vi "BASE-Main.vi"() -> ()   [LabVIEW 2017]
uses:
  <vilib>/Utility/error.llb/DialogType.ctl
  55ed0eea-cd20-493f-8468-85b8c1a0a0c0.vi
panel:
  in  "RECIPE":bool
  out "error out":errorcluster
  in  "Logout":bool
  in  "Stop":bool
  in  "Create Login":bool
  in  "Reports":bool
  in  "Start":bool
  out "Time":string
  out "Date":string
  in  "Login":bool
  # "USB CONNECTOR TESTING"
types:
  T1 = enum8{"Enabled", "Disabled", "Disabled and Grayed Out"}
  T2 = typedef "DialogType.ctl" = u16
  T3 = enum32{"Invalid", "Standard", "Closed", "Hidden", "Minimized", "Maximized"}
  T4 = enum32{"invalid app kind", "Development System", "Run Time System", "Student Edition", "Embedded LabVIEW", "Evaluation", "Custom"}
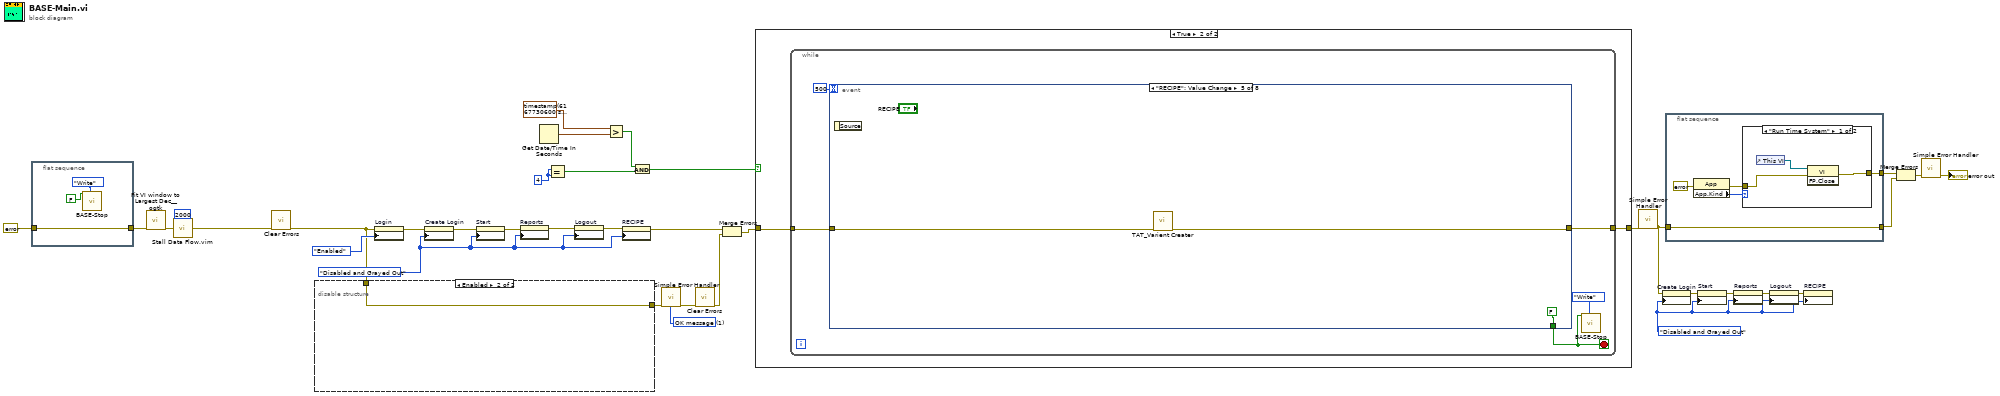
[diagram p0: block diagram]
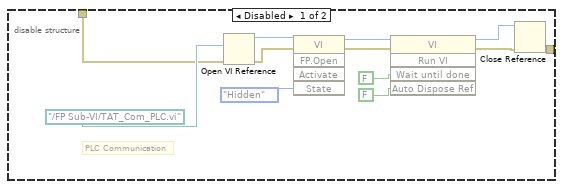
[diagram p2: hidden frame]
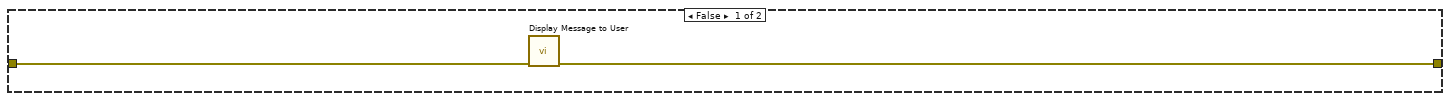
[diagram p4: hidden frame]
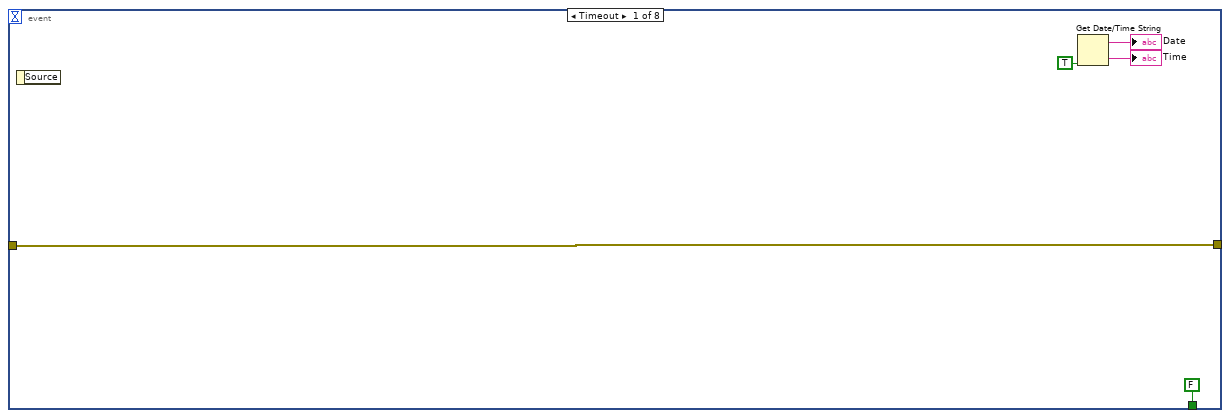
[diagram p5: hidden frame]
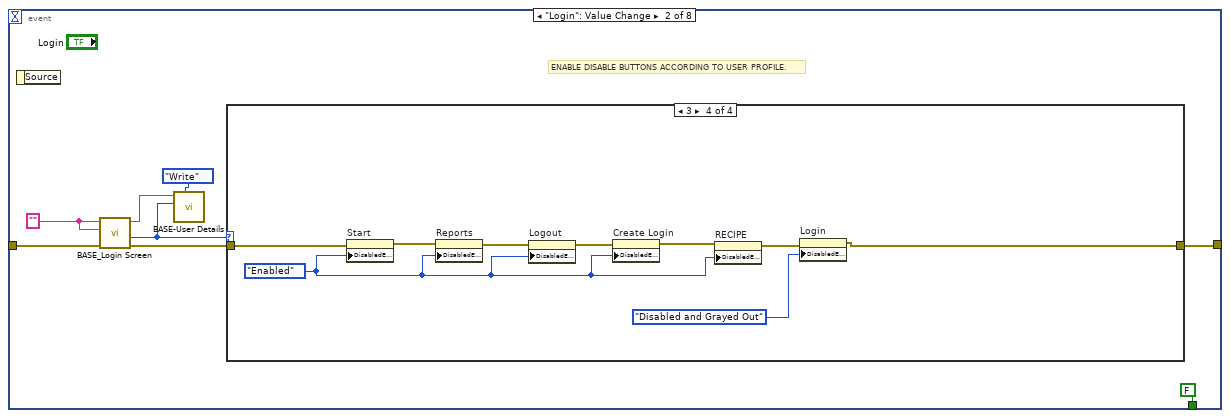
[diagram p6: hidden frame]
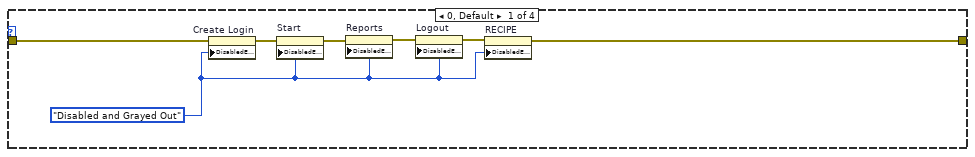
[diagram p7: hidden frame]
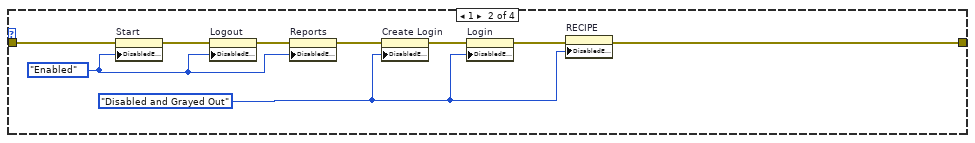
[diagram p8: hidden frame]
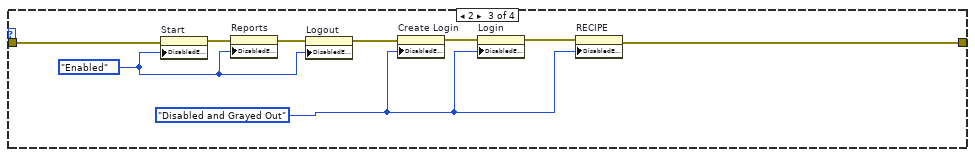
[diagram p9: hidden frame]
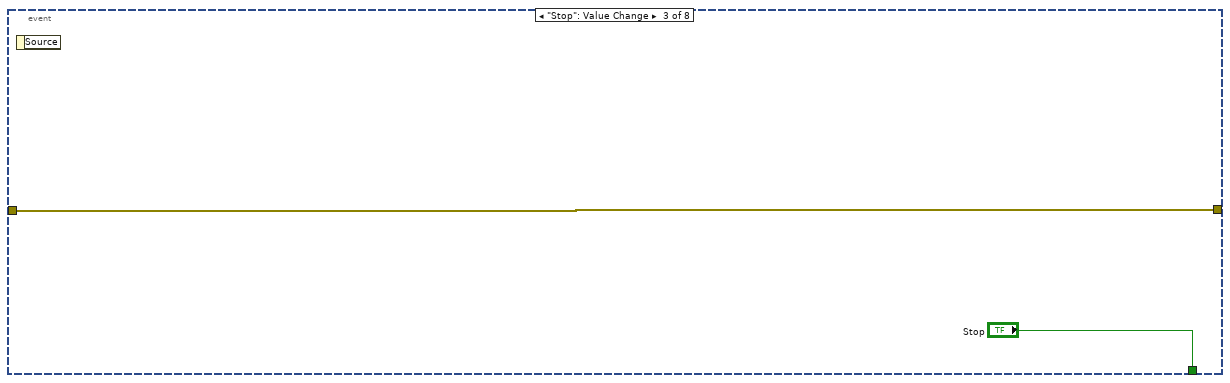
[diagram p10: hidden frame]
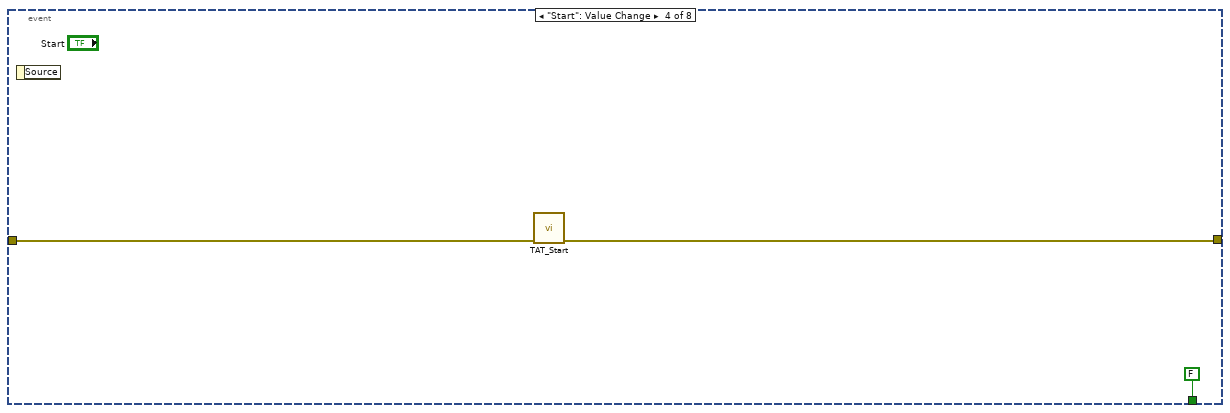
[diagram p11: hidden frame]
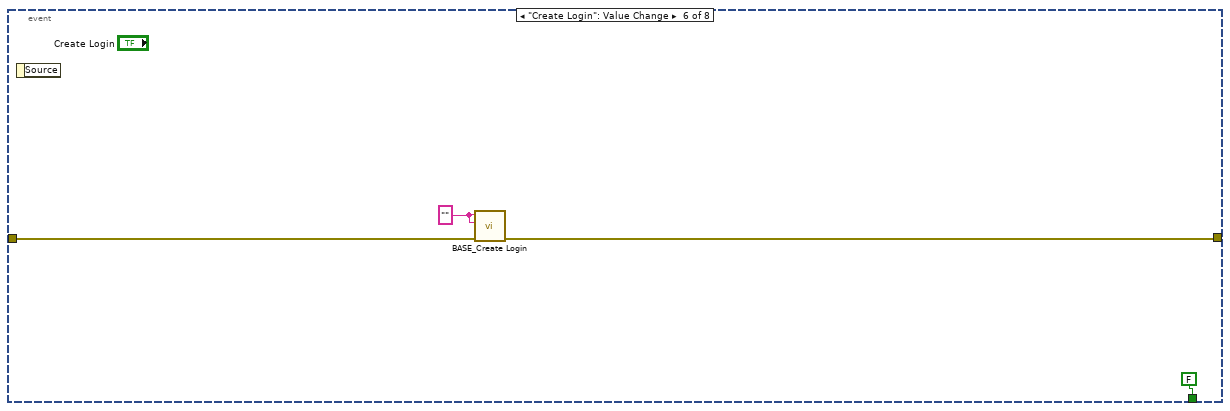
[diagram p12: hidden frame]
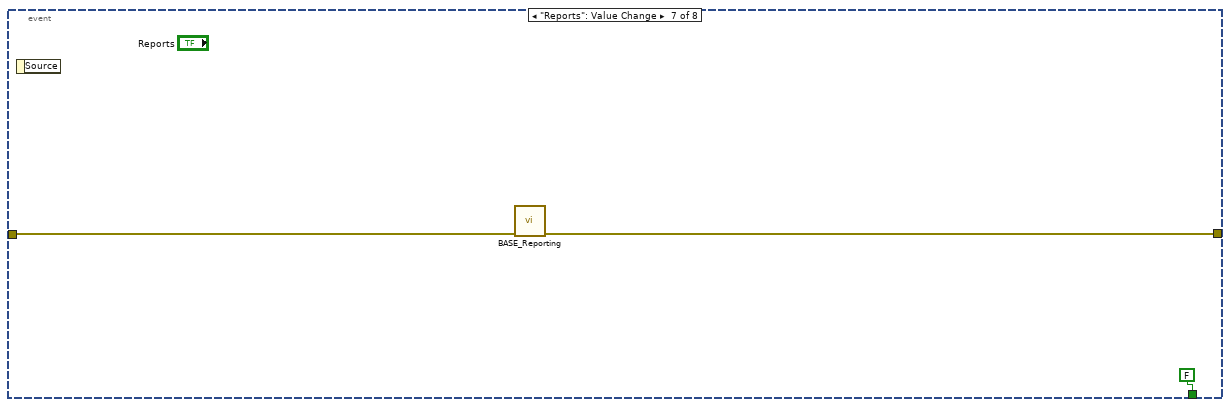
[diagram p13: hidden frame]
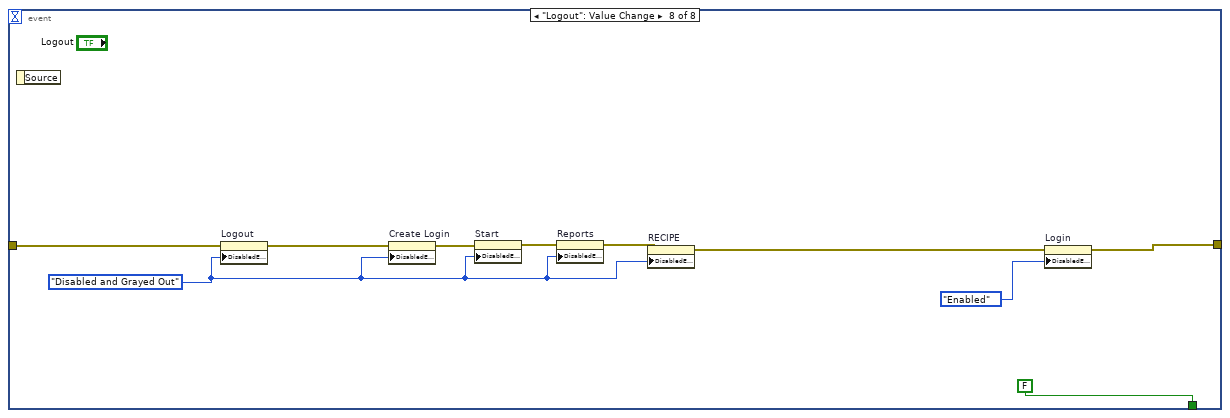
[diagram p14: hidden frame]
diagram:
  w8 = T1."Disabled and Grayed Out" ("Disabled")
  w1 = 4 ("y")
  w24 = T2 1 items=["no dialog", "OK message", "continue or stop message", "OK message + warnings", "continue/stop + warnings"] ("type of dialog (OK msg:1)")
  w9 = T1."Disabled and Grayed Out" ("Disabled")
  n1 = flat-sequence {
    tunnel: [w39] -> w27
    tunnel: errorcluster {"status"=FALSE, "code"=0, "source"=""} ("error constant") -> [w39]
    frame #0 {
      n2 = call "BASE-Stop.vi"("Enum"=enum16{"Read", "Write"}."Write", "Stop"=FALSE) -> ()  [unwired: 9 in, 1 out]
    }
  }
  n3 = call <userlib>:"Fit VI window to Largest Dec__ogtk.vi"("error in (no error)"=w27) -> ("error out"=w14:errorcluster)  [unwired: 5 in, 1 out]
  n4 = call "Stall Data Flow.vim"("value in"=w14, "milliseconds to wait"=u32 2000) -> ("value out"=w13:errorcluster)  [unwired: 1 out]
  n5 = call <vilib>:"Clear Errors.vi"("error in (no error)"=w13) -> ("error out"=w20:errorcluster)  [unwired: 5 in, 1 out]
  n6 = disable-structure shown="Enabled" {
    disable-tunnel: [w41 w52] -> w25
    disable-tunnel: w20 -> [w40 w52]
    frame Disabled {
      # "PLC Communication"
      n7 = Open VI Reference(vi path=path "../FP Sub-VI/TAT_Com_PLC.vi", error in (no error)=w40) -> (vi reference=w48:refnum<vi>, error out=w49:errorcluster)  [unwired: 4 in]
      n8 = invoke class="VI" method="FP.Open"(reference=w48, error in=w49, "State"=T3."Hidden") -> (reference out=w51:refnum<vi>, error out=w50:errorcluster)  [unwired: 2 in, 3 out]
      n9 = invoke class="VI" method="Run VI"(reference=w51, error in=w50, "Wait until done"=FALSE ("Wait Until Done"), "Auto Dispose Ref"=FALSE ("Auto Dispose Reference")) -> (reference out=w47:refnum<vi>, error out=w46:errorcluster)  [unwired: 1 in, 3 out]
      n10 = Close Reference(reference=w47, error in (no error)=w46) -> (error out=w41:errorcluster)
    }
    frame Enabled {
    }
  }
  n11 = property on="Login" class="Bool"(error in=w20, "DisabledEnum"=T1."Enabled" ("Disabled")) -> (error out=w31:errorcluster)  [unwired: 1 in, 1 out]
  n12 = property on="Create Login" class="Bool"(error in=w31, "DisabledEnum"=w9) -> (error out=w35:errorcluster)  [unwired: 1 in, 1 out]
  n13 = property on="Start" class="Bool"(error in=w35, "DisabledEnum"=w9) -> (error out=w10:errorcluster)  [unwired: 1 in, 1 out]
  n14 = property on="Reports" class="Bool"(error in=w10, "DisabledEnum"=w9) -> (error out=w29:errorcluster)  [unwired: 1 in, 1 out]
  n15 = Get Date/Time In Seconds() -> (seconds since 1Jan1904=w16:timestamp)
  n16 = Equal?(x=w1, y=w1) -> (x = y?=w19:bool)
  n17 = property on="Logout" class="Bool"(error in=w29, "DisabledEnum"=w9) -> (error out=w11:errorcluster)  [unwired: 1 in, 1 out]
  n18 = Greater?(x=timestamp(6167730600 s since 1904-01-01), y=w16) -> (0:w15:bool)
  n19 = property on="RECIPE" class="Bool"(error in=w11, "DisabledEnum"=w9) -> (error out=w2:errorcluster)  [unwired: 1 in, 1 out]
  n20 = And(x=w15, y=w19) -> (x .and. y?=w18:bool)
  n21 = call <vilib>:"Simple Error Handler.vi"("type of dialog (OK msg:1)"=w24, "error in (no error)"=w25) -> ("error out"=w23:errorcluster)  [unwired: 3 in, 4 out]
  n22 = call <vilib>:"Clear Errors.vi"("error in (no error)"=w23) -> ("error out"=w22:errorcluster)  [unwired: 5 in, 1 out]
  n23 = Merge Errors(w2, w22) -> (w26:errorcluster)
  n24 = case shown="True" w18 {
    tunnel: w26 -> [w54 w56]
    tunnel: [w53 w55] -> w36
    frame False {
      n25 = call "Display Message to User"("error in (no error)"=w54) -> ("error out"=w53:errorcluster)  [unwired: 9 in, 1 out]
    }
    frame True {
      n26 = while {
        tunnel: w56 -> [w60]
        tunnel: [w59] -> w55
        stop <- w57 stop-if-true
        n27 = event shown="[4] \"RECIPE\": Value Change" {
          selector: _ -> [_ _ _ _ _ _ _ _]
          dyn-events: _ -> [_ _ _ _ _ _ _ _]
          timeout: 500 -> [_ _ _ _ _ _ _ _]
          tunnel: w60 -> [w64 w74 w109 w112 w115 w120 w122 w130]
          tunnel: [w64 w67 w109 w111 w114 w119 w121 w131] -> w59
          tunnel: [FALSE ("Stop") FALSE ("Stop") "Stop" FALSE ("Stop") FALSE ("Stop") FALSE ("Stop") FALSE ("Stop") FALSE ("Stop")] -> w57
          event Timeout {
            n28 = event-data() -> ()  [unwired: 1 in, 1 out]
            n29 = Get Date/Time String(want seconds? (F)=TRUE) -> (date string=→"Date":string, time string=→"Time":string)  [unwired: 2 in]
          }
          event "Login": Value Change {
            w70 = "" ("User Name")
            # "ENABLE DISABLE BUTTONS ACCORDING TO USER PROFILE."
            n30 = event-data() -> ()  [unwired: 1 in, 1 out]
            n31 = call "BASE_Login Screen.vi"("Error In"=w74, "Password"=w70, "User Name"=w70) -> ("error out"=w73:errorcluster, "Level"=w68:i32, "User Name Out"=w71:string)  [unwired: 5 in, 1 out]
            n32 = call "BASE-User Details.vi"("Enum"=enum16{"Read", "Write"}."Write", "Level In"=w68, "User Name In"=w71) -> ()  [unwired: 7 in, 2 out]
            n33 = case shown="3" w68 {
              tunnel: w73 -> [w79 w90 w99 w108]
              tunnel: [w75 w82 w91 w100] -> w67
              frame 0, Default {
                w76 = T1."Disabled and Grayed Out" ("Disabled")
                n34 = property on="Create Login" class="Bool"(error in=w79, "DisabledEnum"=w76) -> (error out=w81:errorcluster)  [unwired: 1 in, 1 out]
                n35 = property on="Start" class="Bool"(error in=w81, "DisabledEnum"=w76) -> (error out=w80:errorcluster)  [unwired: 1 in, 1 out]
                n36 = property on="Reports" class="Bool"(error in=w80, "DisabledEnum"=w76) -> (error out=w77:errorcluster)  [unwired: 1 in, 1 out]
                n37 = property on="Logout" class="Bool"(error in=w77, "DisabledEnum"=w76) -> (error out=w78:errorcluster)  [unwired: 1 in, 1 out]
                n38 = property on="RECIPE" class="Bool"(error in=w78, "DisabledEnum"=w76) -> (error out=w75:errorcluster)  [unwired: 1 in, 1 out]
              }
              frame 1 {
                w84 = T1."Disabled and Grayed Out" ("Disabled")
                w83 = T1."Enabled" ("Disabled")
                n39 = property on="Start" class="Bool"(error in=w90, "DisabledEnum"=w83) -> (error out=w86:errorcluster)  [unwired: 1 in, 1 out]
                n40 = property on="Logout" class="Bool"(error in=w86, "DisabledEnum"=w83) -> (error out=w88:errorcluster)  [unwired: 1 in, 1 out]
                n41 = property on="Reports" class="Bool"(error in=w88, "DisabledEnum"=w83) -> (error out=w89:errorcluster)  [unwired: 1 in, 1 out]
                n42 = property on="Create Login" class="Bool"(error in=w89, "DisabledEnum"=w84) -> (error out=w87:errorcluster)  [unwired: 1 in, 1 out]
                n43 = property on="Login" class="Bool"(error in=w87, "DisabledEnum"=w84) -> (error out=w85:errorcluster)  [unwired: 1 in, 1 out]
                n44 = property on="RECIPE" class="Bool"(error in=w85, "DisabledEnum"=w84) -> (error out=w82:errorcluster)  [unwired: 1 in, 1 out]
              }
              frame 2 {
                w92 = T1."Disabled and Grayed Out" ("Disabled")
                w93 = T1."Enabled" ("Disabled")
                n45 = property on="Start" class="Bool"(error in=w99, "DisabledEnum"=w93) -> (error out=w96:errorcluster)  [unwired: 1 in, 1 out]
                n46 = property on="Reports" class="Bool"(error in=w96, "DisabledEnum"=w93) -> (error out=w98:errorcluster)  [unwired: 1 in, 1 out]
                n47 = property on="Logout" class="Bool"(error in=w98, "DisabledEnum"=w93) -> (error out=w94:errorcluster)  [unwired: 1 in, 1 out]
                n48 = property on="Create Login" class="Bool"(error in=w94, "DisabledEnum"=w92) -> (error out=w97:errorcluster)  [unwired: 1 in, 1 out]
                n49 = property on="Login" class="Bool"(error in=w97, "DisabledEnum"=w92) -> (error out=w95:errorcluster)  [unwired: 1 in, 1 out]
                n50 = property on="RECIPE" class="Bool"(error in=w95, "DisabledEnum"=w92) -> (error out=w91:errorcluster)  [unwired: 1 in, 1 out]
              }
              frame 3 {
                w101 = T1."Enabled" ("Disabled")
                n51 = property on="Start" class="Bool"(error in=w108, "DisabledEnum"=w101) -> (error out=w103:errorcluster)  [unwired: 1 in, 1 out]
                n52 = property on="Reports" class="Bool"(error in=w103, "DisabledEnum"=w101) -> (error out=w107:errorcluster)  [unwired: 1 in, 1 out]
                n53 = property on="Logout" class="Bool"(error in=w107, "DisabledEnum"=w101) -> (error out=w106:errorcluster)  [unwired: 1 in, 1 out]
                n54 = property on="Create Login" class="Bool"(error in=w106, "DisabledEnum"=w101) -> (error out=w105:errorcluster)  [unwired: 1 in, 1 out]
                n55 = property on="RECIPE" class="Bool"(error in=w105, "DisabledEnum"=w101) -> (error out=w104:errorcluster)  [unwired: 1 in, 1 out]
                n56 = property on="Login" class="Bool"(error in=w104, "DisabledEnum"=T1."Disabled and Grayed Out" ("Disabled")) -> (error out=w100:errorcluster)  [unwired: 1 in, 1 out]
              }
            }
          }
          event "Stop": Value Change {
            n57 = event-data() -> ()  [unwired: 1 in, 1 out]
          }
          event "Start": Value Change {
            n58 = event-data() -> ()  [unwired: 1 in, 1 out]
            n59 = call "TAT_Start.vi"("error In"=w112) -> ("error out"=w111:errorcluster)  [unwired: 10 in]
          }
          event "RECIPE": Value Change {
            n60 = event-data() -> ()  [unwired: 1 in, 1 out]
            n61 = call "TAT_Varient Creater.vi"("error in (no error)"=w115) -> ("error out"=w114:errorcluster)  [unwired: 10 in]
          }
          event "Create Login": Value Change {
            w118 = "" ("User Name")
            n62 = event-data() -> ()  [unwired: 1 in, 1 out]
            n63 = call "BASE_Create Login.vi"("Error In"=w120, "Password"=w118, "User Name"=w118) -> ("error out"=w119:errorcluster)  [unwired: 6 in]
          }
          event "Reports": Value Change {
            n64 = event-data() -> ()  [unwired: 1 in, 1 out]
            n65 = call "BASE_Reporting.vi"("error in (no error)"=w122) -> ("error out"=w121:errorcluster)  [unwired: 10 in]
          }
          event "Logout": Value Change {
            w125 = T1."Disabled and Grayed Out" ("Disabled")
            n66 = event-data() -> ()  [unwired: 1 in, 1 out]
            n67 = property on="Logout" class="Bool"(error in=w130, "DisabledEnum"=w125) -> (error out=w126:errorcluster)  [unwired: 1 in, 1 out]
            n68 = property on="Create Login" class="Bool"(error in=w126, "DisabledEnum"=w125) -> (error out=w133:errorcluster)  [unwired: 1 in, 1 out]
            n69 = property on="Start" class="Bool"(error in=w133, "DisabledEnum"=w125) -> (error out=w132:errorcluster)  [unwired: 1 in, 1 out]
            n70 = property on="Reports" class="Bool"(error in=w132, "DisabledEnum"=w125) -> (error out=w127:errorcluster)  [unwired: 1 in, 1 out]
            n71 = property on="RECIPE" class="Bool"(error in=w127, "DisabledEnum"=w125) -> (error out=w124:errorcluster)  [unwired: 1 in, 1 out]
            n72 = property on="Login" class="Bool"(error in=w124, "DisabledEnum"=T1."Enabled" ("Disabled")) -> (error out=w131:errorcluster)  [unwired: 1 in, 1 out]
          }
        }
        n73 = call "BASE-Stop.vi"("Enum"=enum16{"Read", "Write"}."Write", "Stop"=w57) -> ()  [unwired: 9 in, 1 out]
      }
    }
  }
  n74 = call <vilib>:"Simple Error Handler.vi"("error in (no error)"=w36) -> ("error out"=w3:errorcluster)  [unwired: 4 in, 4 out]
  n75 = property on="Create Login" class="Bool"(error in=w3, "DisabledEnum"=w8) -> (error out=w4:errorcluster)  [unwired: 1 in, 1 out]
  n76 = flat-sequence {
    tunnel: [w135] -> w34
    tunnel: [w134] -> w32
    tunnel: w3 -> [w134]
    frame #0 {
      n77 = property class="App"(error in=errorcluster {"status"=FALSE, "code"=0, "source"=""} ("error in (no error)")) -> (error out=w137:errorcluster, "App.Kind"=w138:T4)  [unwired: 1 in, 1 out]
      n78 = case shown="\"Run Time System\"" w138 {
        tunnel: w137 -> [w140 w142]
        tunnel: [w139 w142] -> w135
        frame "Run Time System" {
          n79 = control-ref of="This VI"() -> (w141:refnum<vi>)
          n80 = invoke class="VI" method="FP.Close"(reference=w141, error in=w140) -> (error out=w139:errorcluster)  [unwired: 1 in, 2 out]
        }
        frame "Development System", Default {
        }
      }
    }
  }
  n81 = property on="Start" class="Bool"(error in=w4, "DisabledEnum"=w8) -> (error out=w7:errorcluster)  [unwired: 1 in, 1 out]
  n82 = property on="Reports" class="Bool"(error in=w7, "DisabledEnum"=w8) -> (error out=w5:errorcluster)  [unwired: 1 in, 1 out]
  n83 = property on="Logout" class="Bool"(error in=w5, "DisabledEnum"=w8) -> (error out=w6:errorcluster)  [unwired: 1 in, 1 out]
  n84 = property on="RECIPE" class="Bool"(error in=w6, "DisabledEnum"=w8) -> ()  [unwired: 1 in, 2 out]
  n85 = Merge Errors(w34, w32) -> (w33:errorcluster)
  n86 = call <vilib>:"Simple Error Handler.vi"("error in (no error)"=w33) -> ("error out"=→"error out":errorcluster)  [unwired: 4 in, 4 out]
